vi "Detect Endian.vi"() -> (5 "Endian":T1)   [LabVIEW 2021, in "DataTypes_CIF_U.lvlib"]
uses:
  DataTypes_CIF_U.lvlib
  Endian.ctl
  9c6afb01-b673-4ef1-adb6-e5bb00f5f1bc.vi/c28b0ead-42ad-4072-80a2-aca7f2bd7ce3.vi
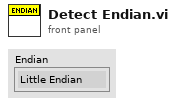
[diagram p1: front panel]
types:
  T1 = typedef "DataTypes_CIF_U.lvlib/Endian.ctl" = enum16{"Little Endian", "Big Endian"}
  T2 = enum16{"big-endian, network order", "native, host order", "little-endian"}
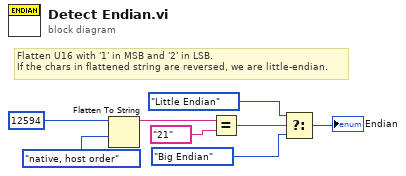
[diagram p0: block diagram]
diagram:
  # "Flatten U16 with '1' in MSB and '2' in LSB.\nIf the chars in flattened string are reversed, we are little-endian."
  n1 = Flatten To String(anything=i16 12594, byte order (0:big-endian, network order)=T2."native, host order") -> (data string=w2:string)  [unwired: 1 in, 3 out]
  n2 = Equal?(x=w2, y="21") -> (x = y?=w1:bool)
  n3 = Select(t=Endian."Little Endian" ("Endian"), s=w1, f=Endian."Big Endian" ("Endian")) -> (s? t:f=→"Endian":T1)
